vi "IndexesCalculate.vi"(10 "j":i32, 11 "i":i32) -> (0 "j_l":i32, 1 "j*":i32, 2 "i_l":i32, 3 "i*":i32)   [LabVIEW 2020]
doc: "Calculate indexes to take subarray for \"Moore neighborhood\"."
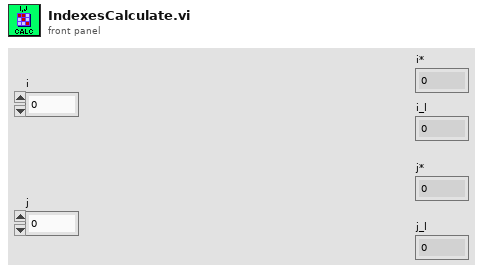
[diagram p1: front panel]
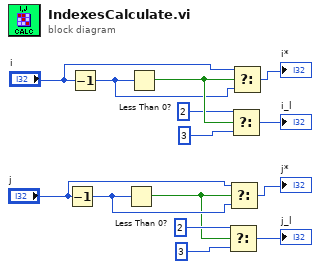
[diagram p0: block diagram]
diagram:
  n1 = Decrement(x="j") -> (x-1=w7:i32)
  n2 = Decrement(x="i") -> (x-1=w12:i32)
  n3 = Less Than 0?(x=w7) -> (x < 0?=w6:bool)
  n4 = Less Than 0?(x=w12) -> (x < 0?=w14:bool)
  n5 = Select(t=2, s=w6, f=3) -> (s? t:f=→"j_l":i32)
  n6 = Select(t="j", s=w6, f=w7) -> (s? t:f=→"j*":i32)
  n7 = Select(t=2, s=w14, f=3) -> (s? t:f=→"i_l":i32)
  n8 = Select(t="i", s=w14, f=w12) -> (s? t:f=→"i*":i32)
